vi "Read Bootloader Software Version.vi"(6 "error in":errorcluster, 8 "MaxRead":i32, 9 "Channel in":u16) -> (0 "error out":errorcluster, 1 "Messages":T1(array[cluster]), 2 "Pass":bool, 3 "Channel out":u16, 4 "Bootloader Version":string)   [LabVIEW 2023]
uses:
  4f930f32-d09a-43ef-bca1-8b214b378bd5.vi
  e8470de1-fa2d-4ee3-b50e-96bd89dc731f.vi
  d0f02419-cfb7-4a5e-bc3c-f035efdb0e96.vi
  Communication/PCAN2023/PCAN API.lvlib
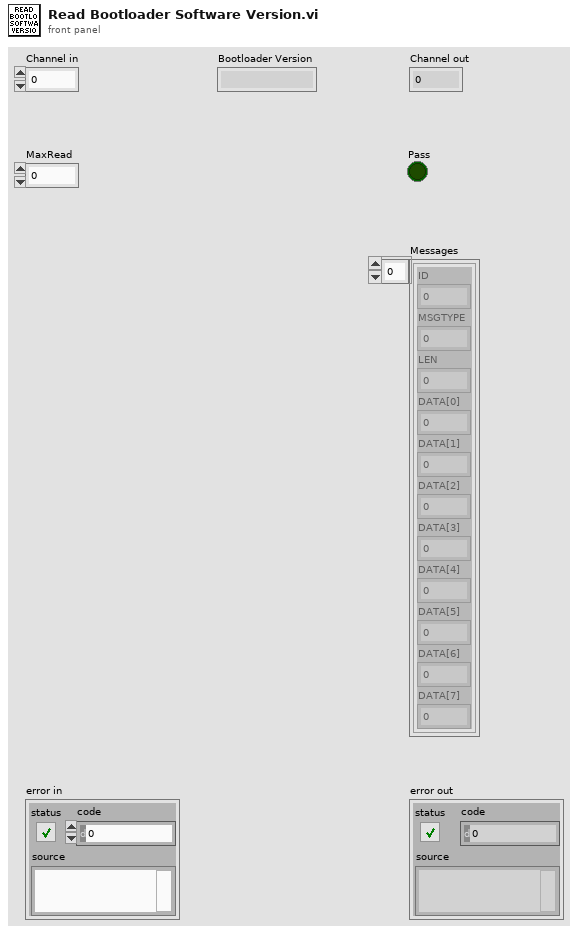
[diagram p1: front panel]
types:
  T1 = cluster{"ID":u32, "MSGTYPE":u8, "LEN":u8, "DATA[0]":u8, "DATA[1]":u8, "DATA[2]":u8, "DATA[3]":u8, "DATA[4]":u8, "DATA[5]":u8, "DATA[6]":u8, "DATA[7]":u8}[]
  T2 = cluster{"ID":u32, "MSGTYPE":u8, "LEN":u8, "DATA[0]":u8, "DATA[1]":u8, "DATA[2]":u8, "DATA[3]":u8, "DATA[4]":u8, "DATA[5]":u8, "DATA[6]":u8, "DATA[7]":u8}
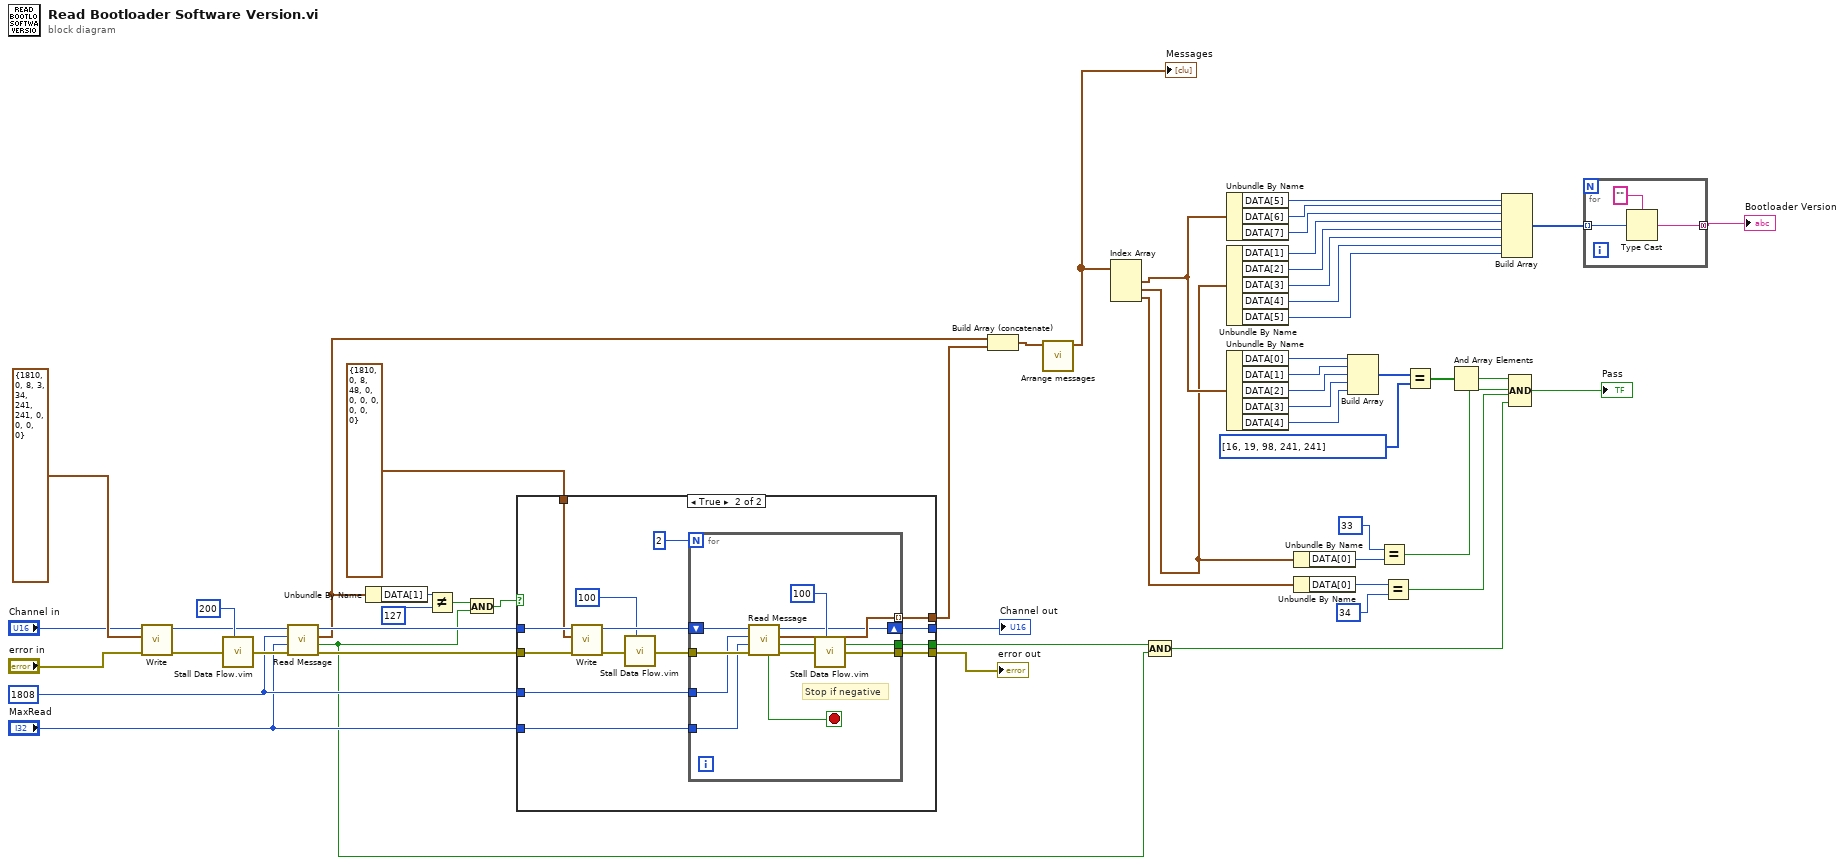
[diagram p0: block diagram]
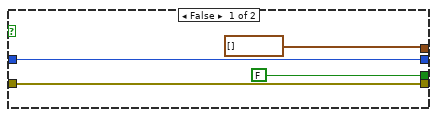
[diagram p2: hidden frame]
diagram:
  (unwired) u32 200 ("milliseconds to wait")
  w10 = u32 1808 ("ID")
  n1 = call "Write.vi"("error in"="error in", "MessageBuffer"=T2 {"ID"=1810, "MSGTYPE"=0, "LEN"=8, "DATA[0]"=3, "DATA[1]"=34, "DATA[2]"=241, "DATA[3]"=241, "DATA[4]"=0, "DATA[5]"=0, "DATA[6]"=0, "DATA[7]"=0}, "Channel"="Channel in") -> ("error out"=w50:errorcluster, "Channel out"=w15:u16)  [unwired: 5 in, 2 out]
  n2 = call "Stall Data Flow.vim"("value in"=w50, "milliseconds to wait"=u32 200) -> ("value out"=w13:errorcluster)  [unwired: 1 out]
  n3 = call "Read Message.vi"("error in"=w13, "MaxRead"="MaxRead", "ID"=w10, "Channel in"=w15) -> ("error out"=w12:errorcluster, "Passed"=w6:bool, "Last Message"=w11:T2, "Channel out"=w14:u16)  [unwired: 3 in, 1 out]
  n4 = Unbundle By Name(w11) -> ("DATA[1]"=w45:u8)
  n5 = Not Equal?(x=w45, y=u8 127) -> (x != y?=w8:bool)
  n6 = And(x=w8, y=w6) -> (x .and. y?=w7:bool)
  n7 = case shown="True" w7 {
    tunnel: w14 -> [w57 w72]
    tunnel: w12 -> [w55 w71]
    tunnel: [w55 w70] -> w49
    tunnel: [FALSE w69] -> w48
    tunnel: [w57 w67] -> w47
    tunnel: T2 {"ID"=1810, "MSGTYPE"=0, "LEN"=8, "DATA[0]"=48, "DATA[1]"=0, "DATA[2]"=0, "DATA[3]"=0, "DATA[4]"=0, "DATA[5]"=0, "DATA[6]"=0, "DATA[7]"=0} ("MessageBuffer") -> [_ w65]
    tunnel: [T1 [] w61] -> w18
    tunnel: w10 -> [_ w60]
    tunnel: "MaxRead" -> [_ w59]
    frame False {
    }
    frame True {
      n8 = call "Write.vi"("error in"=w71, "MessageBuffer"=w65, "Channel"=w72) -> ("error out"=w62:errorcluster, "Channel out"=w68:u16)  [unwired: 5 in, 2 out]
      n9 = call "Stall Data Flow.vim"("value in"=w62, "milliseconds to wait"=u32 100) -> ("value out"=w66:errorcluster)  [unwired: 1 out]
      n10 = for {
        N: 2 -> [_]
        tunnel: [w80] -> w69
        shift-right: [w76] -> w67
        shift-left: w68 -> [w75]
        tunnel: w66 -> [w78]
        tunnel: [w83] -> w70
        tunnel: [w77] -> w61 mode=indexing
        tunnel: w60 -> [w74]
        tunnel: w59 -> [w73]
        stop <- w81 stop-if-true
        # "Stop if negative"
        n11 = call "Read Message.vi"("error in"=w78, "MaxRead"=w73, "ID"=w74, "Channel in"=w75) -> ("error out"=w79:errorcluster, "Passed"=w80:bool, "Last Message"=w77:T2, "Channel out"=w76:u16, "Negative"=w81:bool)  [unwired: 3 in]
        n12 = call "Stall Data Flow.vim"("value in"=w79, "milliseconds to wait"=u32 100) -> ("value out"=w83:errorcluster)  [unwired: 1 out]
      }
    }
  }
  "error out" <- w49
  "Channel out" <- w47
  n13 = Build Array (concatenate)(w11, w18) -> (w5:T1)
  n14 = call "Arrange messages.vi"("Array in"=w5) -> ("Array out"=w4:T1)  [unwired: 10 in]
  "Messages" <- w4
  n15 = Index Array(array=w4) -> (element #1=w3:T2, element #2=w2:T2, element #3=w1:T2)  [unwired: 3 in]
  n16 = Compound Arithmetic op=AND(w48, w6) -> (w16:bool)
  n17 = Unbundle By Name(w3) -> ("DATA[5]"=w28:u8, "DATA[6]"=w27:u8, "DATA[7]"=w26:u8)
  n18 = Unbundle By Name(w2) -> ("DATA[1]"=w23:u8, "DATA[2]"=w22:u8, "DATA[3]"=w21:u8, "DATA[4]"=w20:u8, "DATA[5]"=w19:u8)
  n19 = Unbundle By Name(w3) -> ("DATA[0]"=w43:u8, "DATA[1]"=w42:u8, "DATA[2]"=w41:u8, "DATA[3]"=w40:u8, "DATA[4]"=w39:u8)
  n20 = Unbundle By Name(w2) -> ("DATA[0]"=w36:u8)
  n21 = Unbundle By Name(w1) -> ("DATA[0]"=w33:u8)
  n22 = Build Array(w43, w42, w41, w40, w39) -> (w38:u8[])
  n23 = Equal?(x=u8 33, y=w36) -> (x = y?=w31:bool)
  n24 = Equal?(x=w33, y=u8 34 ("x")) -> (x = y?=w29:bool)
  n25 = Equal?(x=w38, y=u8[] [16, 19, 98, 241, 241]) -> (x = y?=w32:bool[])
  n26 = And Array Elements(Boolean array=w32) -> (logical AND=w30:bool)
  n27 = Build Array(w28, w27, w26, w23, w22, w21, w20, w19) -> (w25:u8[])
  n28 = Compound Arithmetic op=AND(w30, w31, w29, w16) -> (→"Pass":bool)
  n29 = for {
    tunnel: w25 -> [w85] mode=indexing
    tunnel: [w84] -> w24 mode=concatenating
    n30 = Type Cast(type="", x=w85) -> (*(type *) &x=w84:string)
  }
  "Bootloader Version" <- w24
